vi "Get Pin Simulated.vi"(9 "Valor pin":string, 10 "PIN":i32, 11 "CH":i32) -> (1 "Boolean":bool, 2 "String":string, 3 "String 2":string)   [LabVIEW 2020, in "UI Actor.lvlib" / "UI Actor.lvclass"]
uses:
  UI Actor.lvclass
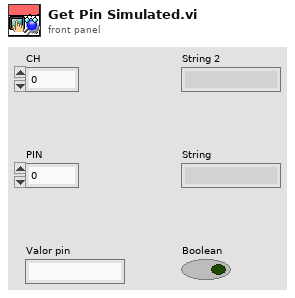
[diagram p1: front panel]
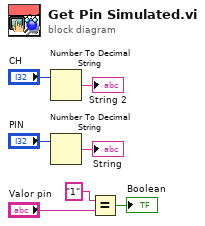
[diagram p0: block diagram]
diagram:
  n1 = Number To Decimal String(number="CH") -> (decimal integer string=→"String 2":string)  [unwired: 1 in]
  n2 = Number To Decimal String(number="PIN") -> (decimal integer string=→"String":string)  [unwired: 1 in]
  n3 = Equal?(x="1", y="Valor pin") -> (x = y?=→"Boolean":bool)
